vi "Read Command Status.vi"(8 "error in (no error)":errorcluster, 11 "Command in":refnum<class "Command.lvclass">) -> (0 "error out":errorcluster, 2 "Command Status":T1, 3 "Command out":refnum<class "Command.lvclass">)   [LabVIEW 2013, in "Robot Actors.lvlib" / "Command.lvlib" / "Command.lvclass"]
uses:
  Command.lvclass
  Command Status.ctl
  Command States.ctl
  Command.lvclass/Command.ctl
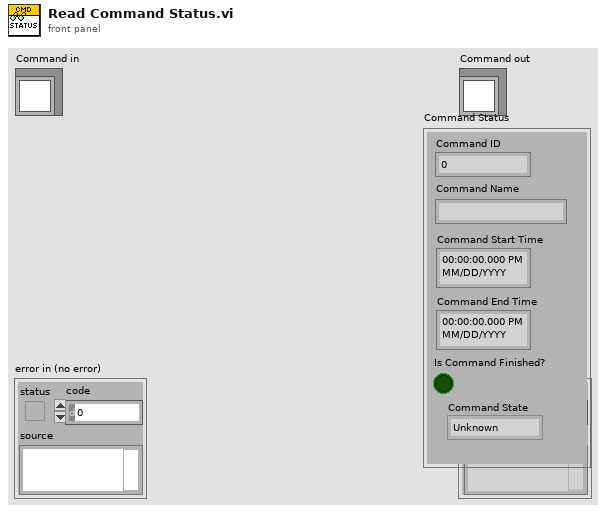
[diagram p1: front panel]
types:
  T1 = typedef "Robot Actors.lvlib/Command.lvlib/Command.lvclass/Command Status.ctl" = cluster{"Command Name":string, "Command Start Time":timestamp, "Command End Time":timestamp, "Is Command Finished?":bool, "Command ID":dbl, "Command State":T2}
  T2 = typedef "Robot Actors.lvlib/Command.lvlib/Command.lvclass/Command States.ctl" = enum16{"Unknown", "Started", "Stopped", "Finished"}
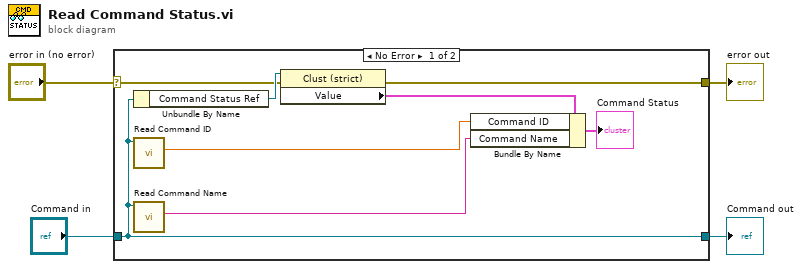
[diagram p0: block diagram]
diagram:
  n1 = case shown="No Error" "error in (no error)" {
    selector: "error in (no error)" -> [w10 w14]
    tunnel: [w9 w14] -> w3
    tunnel: [w6 w13] -> w1
    tunnel: "Command in" -> [w6 w13]
    frame No Error {
      n2 = Unbundle By Name(w6) -> ("Command Status Ref"=w12:refnum<vi>)
      n3 = call-dynamic "Read Command ID.vi"("Command in"=w6) -> ("Command ID"=w7:dbl)  [unwired: 8 in, 2 out]
      n4 = call-dynamic "Read Command Name.vi"("Command in"=w6) -> ("Command Name"=w5:string)  [unwired: 8 in, 2 out]
      n5 = property class="Clust (strict)"(reference=w12, error in=w10) -> (error out=w9:errorcluster, "Value"=w11:T1)  [unwired: 1 out]
      n6 = Bundle By Name(cluster=w11, "Command ID"=w7, "Command Name"=w5) -> (→"Command Status":T1)
    }
    frame Error {
    }
  }
  "error out" <- w3
  "Command out" <- w1
